vi "Write Fecha.vi"(8 "error in (no error)":errorcluster, 10 "Fecha":string, 11 "FirstActor in":refnum<class "FirstActor.lvclass">) -> (0 "error out":errorcluster, 3 "FirstActor out":refnum<class "FirstActor.lvclass">)   [LabVIEW 2020, in "FirstActor.lvlib" / "FirstActor.lvclass"]
uses:
  FirstActor.lvclass
  FirstActor.lvclass/FirstActor.ctl
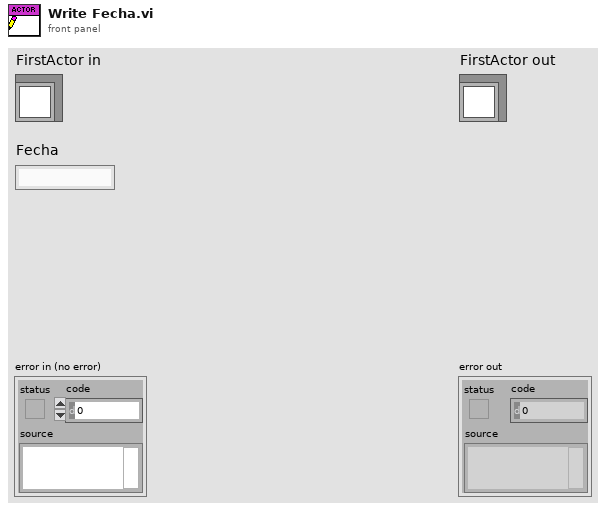
[diagram p1: front panel]
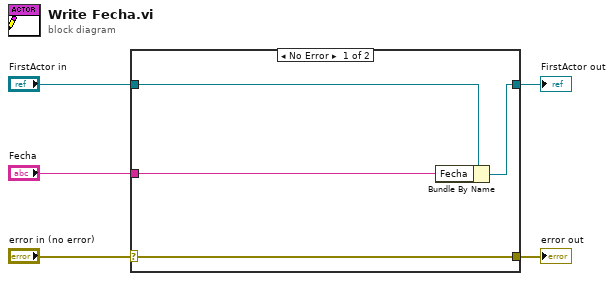
[diagram p0: block diagram]
diagram:
  n1 = case shown="No Error" "error in (no error)" {
    selector: "error in (no error)" -> [w9 w10]
    tunnel: [w9 w10] -> w4
    tunnel: [w7 w11] -> w2
    tunnel: "FirstActor in" -> [w8 w11]
    tunnel: "Fecha" -> [w6 _]
    frame No Error {
      n2 = Bundle By Name(cluster=w8, "Fecha"=w6) -> (w7:refnum<class "FirstActor.lvclass">)
    }
    frame Error {
    }
  }
  "error out" <- w4
  "FirstActor out" <- w2
